vi "Read PID Info.vi"(0 "VISA Session In":refnum<visa-resource-name>="Alicat", 3 "error in":errorcluster, 4 "Unit ID (A)":string="A") -> (7 "VISA Session Out":refnum<visa-resource-name>, 8 "PID Settings":T1={"Valve Amount"=enum."Single Valve", "PID Type"=enum."PDF", "Valve Offset"=15000, "P Gain"=100, "D Gain"=5000, "I Gain"=0}, 10 "error out":errorcluster)   [LabVIEW 2014]
doc: "Returns the PID control algorithm settings: P gain, I gain, D gain, PID loop type, valve offset, and whether the device is a single vale unit or a dual valve unit."
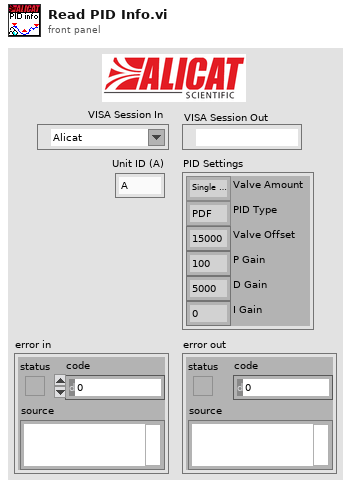
[diagram p1: front panel]
types:
  T1 = cluster{"Valve Amount":enum8{"Single Valve", "Dual Valve"}, "PID Type":enum8{"PDF", "PD2I"}, "Valve Offset":i32, "P Gain":i32, "D Gain":i32, "I Gain":i32}
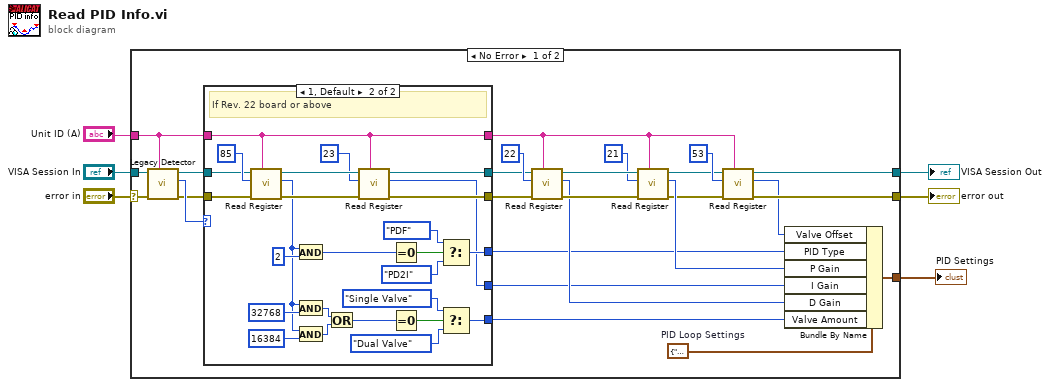
[diagram p0: block diagram]
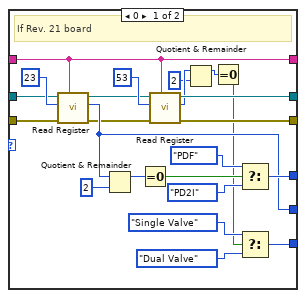
[diagram p2: hidden frame]
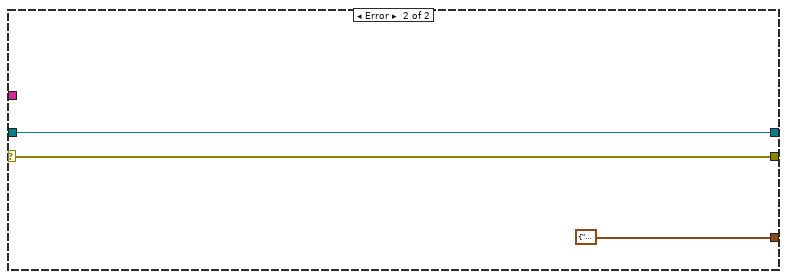
[diagram p3: hidden frame]
diagram:
  n1 = case shown="No Error" "error in" {
    selector: "error in" -> [w17 w83]
    tunnel: [w13 w83] -> w6
    tunnel: [w10 w84] -> w5
    tunnel: "VISA Session In" -> [w28 w84]
    tunnel: "Unit ID (A)" -> [w22 _]
    tunnel: [w19 T1 {"Valve Amount"=enum."Single Valve", "PID Type"=enum."PDF", "Valve Offset"=0, "P Gain"=0, "D Gain"=0, "I Gain"=0} ("PID Loop Settings")] -> w1
    frame No Error {
      w8 = T1 {"Valve Amount"=enum."Single Valve", "PID Type"=enum."PD2I", "Valve Offset"=0, "P Gain"=0, "D Gain"=0, "I Gain"=0}  # PID Loop Settings
      n2 = call "Legacy Detector.vi"("Unit ID (A)"=w22, "error in"=w17, "VISA Session In"=w28) -> ("error out"=w25:errorcluster, "Legacy Status"=w27:u8, "VISA Session Out"=w26:refnum<visa-resource-name>)  [unwired: 6 in]
      n3 = case shown="1, Default" w27 {
        tunnel: w26 -> [w54 w77]
        tunnel: w25 -> [w53 w76]
        tunnel: [w43 w75] -> w24
        tunnel: [w44 w74] -> w23
        tunnel: w22 -> [w40 w73]
        tunnel: [w40 w73] -> w9
        tunnel: [w46 w61] -> w16
        tunnel: [w49 w69] -> w18
        tunnel: [w37 w56] -> w15
        frame 0 {
          # "If Rev. 21 board"
          n4 = call "Read Register.vi"("Unit ID (A)"=w40, "error in"=w53, "Register address"=u16 23, "VISA Session In"=w54) -> ("error out"=w42:errorcluster, "Register Value (I32)"=w46:i32, "VISA Session Out"=w41:refnum<visa-resource-name>)  [unwired: 5 in]
          n5 = Quotient & Remainder(x=w46, y=2) -> (x-y*floor(x/y)=w51:i32)  [unwired: 1 out]
          n6 = Equal To 0?(x=w51) -> (x = 0?=w50:bool)
          n7 = call "Read Register.vi"("Unit ID (A)"=w40, "error in"=w42, "Register address"=u16 53, "VISA Session In"=w41) -> ("error out"=w43:errorcluster, "Register Value (I32)"=w39:i32, "VISA Session Out"=w44:refnum<visa-resource-name>)  [unwired: 5 in]
          n8 = Quotient & Remainder(x=w39, y=2) -> (x-y*floor(x/y)=w33:i32)  [unwired: 1 out]
          n9 = Equal To 0?(x=w33) -> (x = 0?=w34:bool)
          n10 = Select(t=enum8{"PDF", "PD2I"}."PDF" ("PID Type"), s=w50, f=enum8{"PDF", "PD2I"}."PD2I" ("PID Type")) -> (s? t:f=w49:enum8{"PDF", "PD2I"})
          n11 = Select(t=enum8{"Single Valve", "Dual Valve"}."Single Valve" ("Valve Amount"), s=w34, f=enum8{"Single Valve", "Dual Valve"}."Dual Valve" ("Valve Amount")) -> (s? t:f=w37:enum8{"Single Valve", "Dual Valve"})
        }
        frame 1, Default {
          # "If Rev. 22 board or above"
          n12 = call "Read Register.vi"("Unit ID (A)"=w73, "error in"=w76, "Register address"=u16 85 ("register"), "VISA Session In"=w77) -> ("error out"=w79:errorcluster, "Register Value (I32)"=w63:i32, "VISA Session Out"=w80:refnum<visa-resource-name>)  [unwired: 5 in]
          n13 = And(x=w63, y=2) -> (x .and. y?=w62:i32)
          n14 = And(x=w63, y=32768) -> (x .and. y?=w66:i32)
          n15 = And(x=w63, y=16384) -> (x .and. y?=w65:i32)
          n16 = Or(x=w66, y=w65) -> (x .or. y?=w57:i32)
          n17 = call "Read Register.vi"("Unit ID (A)"=w73, "error in"=w79, "Register address"=u16 23, "VISA Session In"=w80) -> ("error out"=w75:errorcluster, "Register Value (I32)"=w61:i32, "VISA Session Out"=w74:refnum<visa-resource-name>)  [unwired: 5 in]
          n18 = Equal To 0?(x=w62) -> (x = 0?=w70:bool)
          n19 = Equal To 0?(x=w57) -> (x = 0?=w60:bool)
          n20 = Select(t=enum8{"PDF", "PD2I"}."PDF" ("PID Type"), s=w70, f=enum8{"PDF", "PD2I"}."PD2I" ("PID Type")) -> (s? t:f=w69:enum8{"PDF", "PD2I"})
          n21 = Select(t=enum8{"Single Valve", "Dual Valve"}."Single Valve" ("Valve Amount"), s=w60, f=enum8{"Single Valve", "Dual Valve"}."Dual Valve" ("Valve Amount")) -> (s? t:f=w56:enum8{"Single Valve", "Dual Valve"})
        }
      }
      n22 = call "Read Register.vi"("Unit ID (A)"=w9, "error in"=w24, "Register address"=u16 22, "VISA Session In"=w23) -> ("error out"=w31:errorcluster, "Register Value (I32)"=w21:i32, "VISA Session Out"=w32:refnum<visa-resource-name>)  [unwired: 5 in]
      n23 = call "Read Register.vi"("Unit ID (A)"=w9, "error in"=w31, "Register address"=u16 21, "VISA Session In"=w32) -> ("error out"=w12:errorcluster, "Register Value (I32)"=w20:i32, "VISA Session Out"=w11:refnum<visa-resource-name>)  [unwired: 5 in]
      n24 = call "Read Register.vi"("Unit ID (A)"=w9, "error in"=w12, "Register address"=u16 53, "VISA Session In"=w11) -> ("error out"=w13:errorcluster, "Register Value (I32)"=w7:i32, "VISA Session Out"=w10:refnum<visa-resource-name>)  [unwired: 5 in]
      n25 = Bundle By Name(cluster=w8, "Valve Offset"=w7, "PID Type"=w18, "P Gain"=w20, "I Gain"=w16, "D Gain"=w21, "Valve Amount"=w15) -> (w19:T1)
    }
    frame Error {
    }
  }
  "error out" <- w6
  "VISA Session Out" <- w5
  "PID Settings" <- w1
